vi "Config File Builder UI.vi"() -> ()   [LabVIEW 2016]
uses:
  UI Mode.ctl
  <vilib>/Utility/sysdir.llb/System Directory Type.ctl
  <vilib>/Utility/config.llb/Write Key (String).vi
  <vilib>/Utility/config.llb/NI_LVConfig.lvlib
panel:
  out "error out":errorcluster
  in  "UI Mode":T1
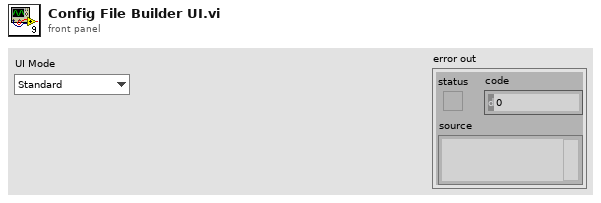
[diagram p1: front panel]
types:
  T1 = typedef "UI Mode.ctl" = enum16{"Standard", "Hidden"}
  T2 = typedef "System Directory Type.ctl" = i32
  T3 = typedef "NI_LVConfig.lvlib/Config Data RefNum.ctl" = refnum<k1>
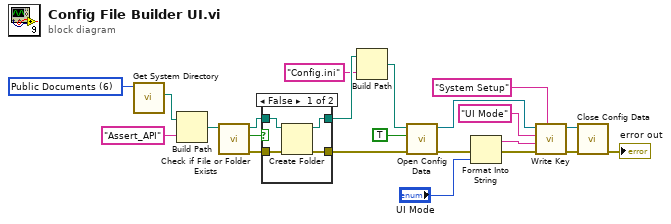
[diagram p0: block diagram]
diagram:
  w21 = T2 6 items=["User Home"=0, "User Desktop"=1, "User Documents"=2, "User Application Data"=3, "User Preferences"=4, "User Temporary"=5, "Public Documents"=6, "Public Application Data"=7, "Public Preferences"=8, "Public Cache"=13, "System Core Libraries"=9, "System Installed Libraries"=10, "Application Files"=11, "Boot Volume Root"=12] ("system directory type")
  n1 = call <vilib>:"Get System Directory.vi"("system directory type"=w21) -> ("system directory"=w20:path)  [unwired: 10 in]
  n2 = Build Path(base path=w20, name or relative path="Assert_API") -> (appended path=w8:path)
  n3 = call <vilib>:"Check if File or Folder Exists.vi"("path"=w8) -> ("error out"=w5:errorcluster, "file or folder exists?"=w6:bool, "dup path"=w7:path)  [unwired: 8 in]
  n4 = case shown="False" w6 {
    tunnel: w7 -> [w26 w27]
    tunnel: w5 -> [w25 w28]
    tunnel: [w24 w28] -> w4
    tunnel: [w23 w27] -> w3
    frame False {
      n5 = Create Folder(path (use dialog)=w26, error in=w25) -> (created path=w23:path, error out=w24:errorcluster)  [unwired: 1 in, 1 out]
    }
    frame True {
    }
  }
  n6 = Build Path(base path=w3, name or relative path="Config.ini") -> (appended path=w1:path)
  n7 = call <vilib>:"Open Config Data.vi"("error in (no error)"=w4, "create file if necessary (T)"=TRUE, "configuration file path"=w1) -> ("error out"=w11:errorcluster, "refnum"=w17:T3)  [unwired: 6 in, 1 out]
  n8 = Format Into String(error in=w11, "UI Mode") -> (resulting string=w14:string, error out=w10:errorcluster)  [unwired: 2 in]
  n9 = call-poly <vilib>:"Write Key.vi"("section"="System Setup", "error in (no error)"=w10, "value"=w14, "key"="UI Mode", "refnum"=w17) -> ("error out"=w12:errorcluster, "refnum out"=w13:T3)  [unwired: 4 in, 1 out]
  n10 = call <vilib>:"Close Config Data.vi"("error in (no error)"=w12, "refnum"=w13) -> ("error out"=→"error out":errorcluster)  [unwired: 8 in, 1 out]
